vi "Measure_Paste_LED.vi"(8 "error in (no error)":errorcluster, 10 "Parameters":string, 11 "reference in":refnum<class "Test_Flux_Capacitor.lvclass">) -> (0 "error out":errorcluster, 2 "Result":dbl, 3 "reference out":refnum<class "Test_Flux_Capacitor.lvclass">)   [LabVIEW 2022 SP3, in "Test_Flux_Capacitor.lvlib" / "Test_Flux_Capacitor.lvclass"]
uses:
  Test_Flux_Capacitor.lvclass
  ParameterTypes/Paste_LED.ctl
  ParameterTypes/DMM_DCA.ctl
  <vilib>/Analysis/baseanly.llb/Mean (DBL).vi
  Components/SwitchBase.lvlibp/SwitchBase.lvclass
  Components/DMM_Keysight_34980A.lvlibp/DMM_Keysight_34980A.lvclass
  <vilib>/Analysis/NI_AALBase.lvlib
  <vilib>/JDP Science/JSONtext/JSONtext.lvlib
panel:
  in  "Parameter_Type":T1={"Pre_Switch"="", "Post_Switch"="", "Wait (msec)"=0, "Scale"=0.0, "DMM_DCA"={"Range"=enum."Auto", "Resolution"=enum."Default", "Samples"=1, "dt (s)"=0.0, "Timeout (s)"=10000.0}, "Sensor"=enum."1", "DutyCycle%"=0}
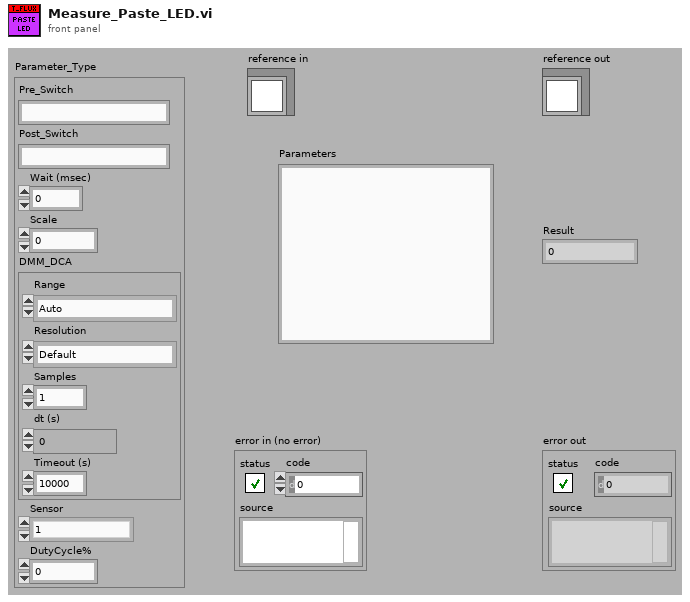
[diagram p1: front panel]
types:
  T1 = typedef "Test_Flux_Capacitor.lvlib/Test_Flux_Capacitor.lvclass/Paste_LED.ctl" = cluster{"Pre_Switch":string, "Post_Switch":string, "Wait (msec)":u32, "Scale":dbl, "DMM_DCA":T2, "Sensor":enum16{"1", "2", "3", "4", "5", "6", "7", "8", "o_large", "o_small"}, "DutyCycle%":u16}
  T2 = typedef "Test_Flux_Capacitor.lvlib/Test_Flux_Capacitor.lvclass/DMM_DCA.ctl" = cluster{"Range":enum16{"10 mA", "100 mA", "1 A", "Auto", "Minimum", "Maximum"}, "Resolution":enum16{"4 1/2", "5 1/2", "6 1/2", "Least", "Highest", "Default"}, "Samples":u32, "dt (s)":dbl, "Timeout (s)":dbl}
  T3 = typedef "Test_Flux_Capacitor.lvlib/Test_Flux_Capacitor.lvclass/ObjectAttributes.ctl" = cluster{"Config":T4, "DMM":refnum<class "DMM_Keysight_34980A.lvclass">, "LCR":refnum<class "LCR_BK891.lvclass">, "PSU":refnum<class "PSU_Base.lvclass">, "Switch_Manager":refnum<class "SwitchBase.lvclass">, "FRAM":string, "Flux_Capacitor":refnum<class "Flux_Capacitor.lvclass">, "Frequency_Counter":refnum<class "Frequency_Counter_Base.lvclass">, "JTAG":refnum<class "JTAG_Base.lvclass">}
  T4 = typedef "Test_Flux_Capacitor.lvlib/Test_Flux_Capacitor.lvclass/Config.ctl" = cluster{"default":string}
  T5 = enum16{"10 mA", "100 mA", "1 A", "Auto", "Minimum", "Maximum"}
  T6 = enum16{"4 1/2", "5 1/2", "6 1/2", "Least", "Highest", "Default"}
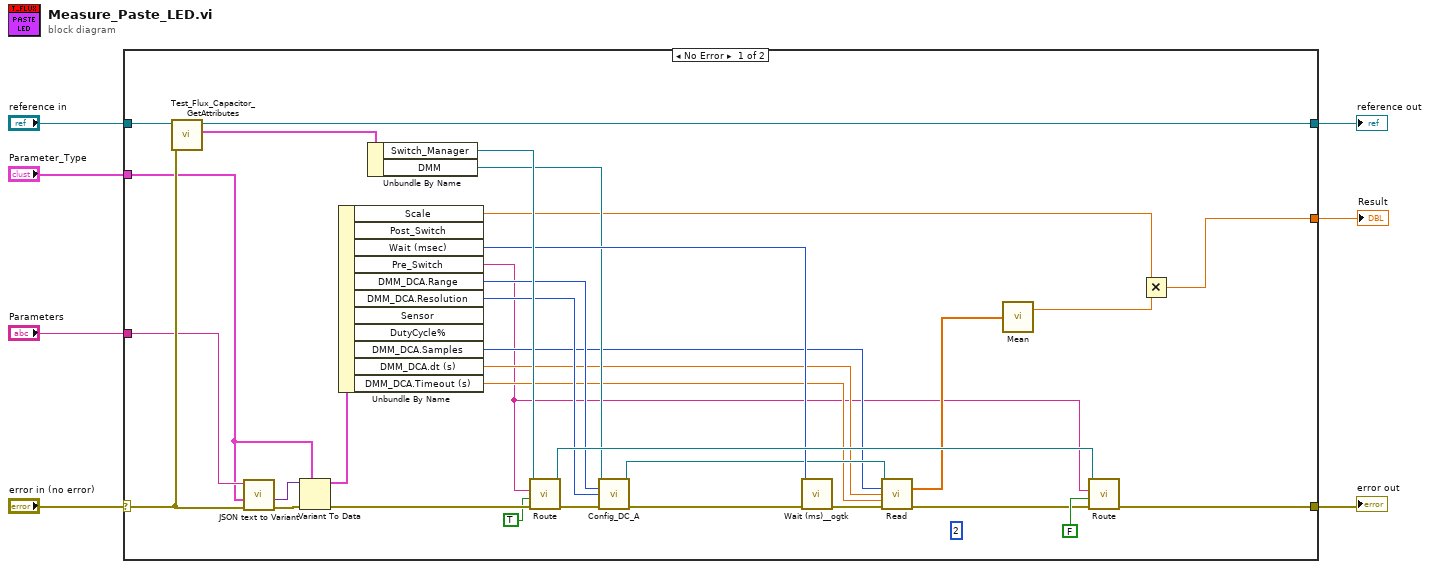
[diagram p0: block diagram]
diagram:
  n1 = case shown="No Error" "error in (no error)" {
    selector: "error in (no error)" -> [w17 w41]
    tunnel: [w33 w41] -> w6
    tunnel: [w38 w40] -> w4
    tunnel: "reference in" -> [w39 w40]
    tunnel: "Parameters" -> [w15 _]
    tunnel: "Parameter_Type" -> [w14 _]
    tunnel: [w18 _] -> w1
    frame No Error {
      (unwired) u16 2 ("DutyCycle%")
      n2 = call "Test_Flux_Capacitor_GetAttributes.vi"("error in (no error)"=w17, "reference in"=w39) -> ("Data"=w37:T3, "reference out"=w38:refnum<class "Test_Flux_Capacitor.lvclass">)  [unwired: 6 in, 2 out]
      n3 = call <vilib>:"JSON text to Variant.vi"("error in (no error)"=w17, "Data Type"=w14, "JSON"=w15) -> ("error out"=w16:errorcluster, "Variant out"=w13:variant)  [unwired: 7 in]
      n4 = Variant To Data(error in=w16, type=w14, Variant=w13) -> (data=w36:T1, error out=w32:errorcluster)
      n5 = Unbundle By Name(w36) -> ("Scale"=w19:dbl, "Wait (msec)"=w31:u32, "Pre_Switch"=w12:string, "DMM_DCA.Range"=w28:T5, "DMM_DCA.Resolution"=w27:T6, "DMM_DCA.Samples"=w24:u32, "DMM_DCA.dt (s)"=w23:dbl, "DMM_DCA.Timeout (s)"=w22:dbl)  [unwired: 3 out]
      n6 = Unbundle By Name(w37) -> ("Switch_Manager"=w35:refnum<class "SwitchBase.lvclass">, "DMM"=w29:refnum<class "DMM_Keysight_34980A.lvclass">)
      n7 = call-dynamic "Route.vi"("error in (no error)"=w32, "Connect"=TRUE, "channel 1"=w12, "reference in"=w35) -> ("error out"=w30:errorcluster, "reference in"=w34:refnum<class "SwitchBase.lvclass">)  [unwired: 6 in]
      n8 = call-dynamic "Config_DC_A.vi"("reference in"=w29, "Range (3:Auto)"=w28, "Resolution (5:Default)"=w27, "error in (no error)"=w30) -> ("reference in"=w25:refnum<class "DMM_Keysight_34980A.lvclass">, "error out"=w8:errorcluster)  [unwired: 10 in]
      n9 = call <userlib>:"Wait (ms)__ogtk.vi"("error in (no error)"=w8, "milliseconds to wait"=w31) -> ("error out"=w26:errorcluster)  [unwired: 8 in, 1 out]
      n10 = call-dynamic "Read.vi"("reference in"=w25, "Samples"=w24, "dt"=w23, "Timeout (10 s)"=w22, "error in (no error)"=w26) -> ("Measurement"=w21:dbl[], "error out"=w9:errorcluster)  [unwired: 7 in, 2 out]
      n11 = call-poly <vilib>:"Mean.vi"("X"=w21) -> ("mean"=w20:dbl)  [unwired: 1 out]
      n12 = call-dynamic "Route.vi"("error in (no error)"=w9, "Connect"=FALSE, "channel 1"=w12, "reference in"=w34) -> ("error out"=w33:errorcluster)  [unwired: 6 in, 1 out]
      n13 = Multiply(x=w19, y=w20) -> (x*y=w18:dbl)
    }
    frame Error {
    }
  }
  "Result" <- w1
  "error out" <- w6
  "reference out" <- w4
